vi "Auth Extra.vi"(8 "error in (no error)":errorcluster, 10 "authextra in":string="{}", 11 "WampCraAuthenticator in":refnum<class "WampCraAuthenticator.lvclass">) -> (0 "error out":errorcluster, 2 "authextra":string caption="authextra out", 3 "WampCraAuthenticator out":refnum<class "WampCraAuthenticator.lvclass">)   [LabVIEW 2020]
uses:
  WampCraAuthenticator.lvclass
  WampCraAuthenticator.lvclass/WampCraAuthenticator.ctl
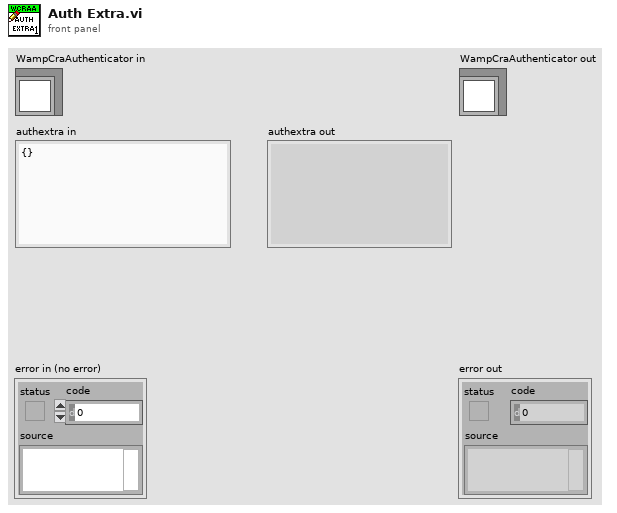
[diagram p1: front panel]
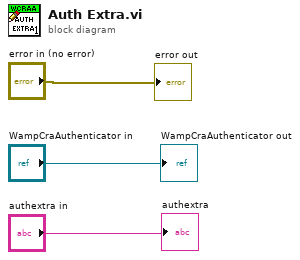
[diagram p0: block diagram]
diagram:
  "error out" <- "error in (no error)"
  "WampCraAuthenticator out" <- "WampCraAuthenticator in"
  "authextra" <- "authextra in"
